vi "Broadcast Map File Path.vi"(8 "error in (no error)":errorcluster, 11 "Yaml Model in":refnum<class "Yaml Model.lvclass">) -> (0 "error out":errorcluster, 3 "Yaml Model out":refnum<class "Yaml Model.lvclass">)   [LabVIEW 2020, in "Yaml Model.lvlib" / "Yaml Model.lvclass"]
uses:
  Yaml Model.lvclass
  Yaml Model Messages/Abstract Map File Path Msg/Abstract Map File Path Msg.lvclass
  C:/Program Files/National Instruments/LabVIEW 2020/vi.lib/ActorFrameworkObserver/Data Message/Data Message.lvclass
  Yaml Model.lvclass/Yaml Model.ctl
  <vilib>/ActorFrameworkObserver/Actor Register/Actor Register.lvclass
panel:
  # "NOTICE -- YOU MUST LEAVE THIS NOTICE IN PLACE.\n\nCopyright (c) 2017, LIANG LIU Shawn.Liu.cn@gmail.com\nAll rights reserved.\n\nRedistribution and use in source and binary forms, with or without modification, are permitted provided that the following conditions are met:\n-Redistributions of source code must retain the above copyright notice, this list of conditions and the following disclaimer.\n-Redistributions in binary form must reproduce the above copyright notice, this list of conditions and the following disclaimer in the documentation and/or other materials provided with the distribution.\n-Neither the name of the eLp nor the names of its contributors may be used to endorse or promote products derived from this software without specific prior written permission.\n\nTHIS SOFTWARE IS PROVIDED BY THE COPYRIGHT HOLDERS AND CONTRIBUTORS \"AS IS\" AND ANY EXPRESS OR IMPLIED WARRANTIES, INCLUDING, BUT NOT LIMITED TO, THE IMPLIED WARRANTIES OF MERCHANTABILITY AND FITNESS FOR A PARTICULAR PURPOSE ARE DISCLAIMED. IN NO EVENT SHALL THE COPYRIGHT HOLDER OR CONTRIBUTORS BE LIABLE FOR ANY DIRECT, INDIRECT, INCIDENTAL, SPECIAL, EXEMPLARY, OR CONSEQUENTIAL DAMAGES (INCLUDING, BUT NOT LIMITED TO, PROCUREMENT OF SUBSTITUTE GOODS OR SERVICES; LOSS OF USE, DATA, OR PROFITS; OR BUSINESS INTERRUPTION) HOWEVER CAUSED AND ON ANY THEORY OF LIABILITY, WHETHER IN CONTRACT, STRICT LIABILITY, OR TORT (INCLUDING NEGLIGENCE OR OTHERWISE) ARISING IN ANY WAY OUT OF THE USE OF THIS SOFTWARE, EVEN IF ADVISED OF THE POSSIBILITY OF SUCH DAMAGE."
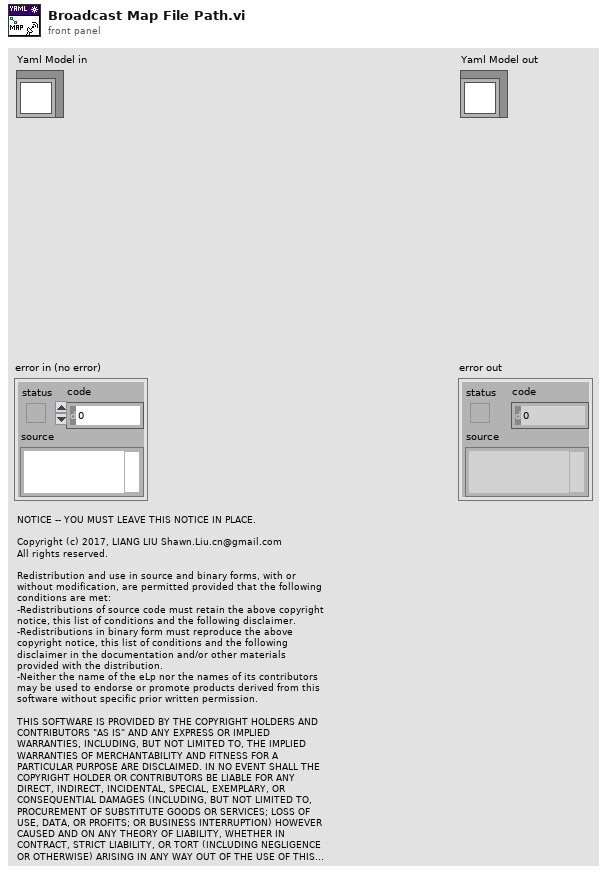
[diagram p1: front panel]
types:
  T1 = cluster{"Image":string, "Resolution":dbl, "Origin":cluster{"X":dbl, "Y":dbl, "R":dbl}, "Occupied Thresh":dbl, "Free Thresh":dbl, "Negate":bool}
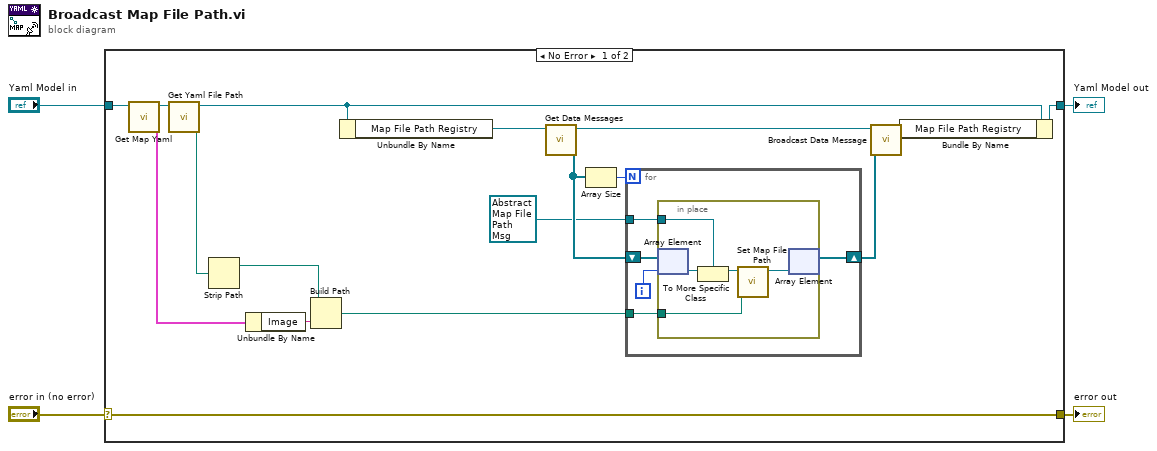
[diagram p0: block diagram]
diagram:
  n1 = case shown="No Error" "error in (no error)" {
    selector: "error in (no error)" -> [w19 w33]
    tunnel: "Yaml Model in" -> [w21 w32]
    tunnel: [w20 w32] -> w3
    tunnel: [w19 w33] -> w1
    frame No Error {
      n2 = call "Get Map Yaml.vi"("Yaml Model in"=w21) -> ("Map Yaml"=w14:T1, "Yaml Model out"=w18:refnum<class "Yaml Model.lvclass">)  [unwired: 9 in]
      n3 = call "Get Yaml File Path.vi"("Yaml Model in"=w18) -> ("Yaml File Path"=w16:path, "Yaml Model out"=w17:refnum<class "Yaml Model.lvclass">)  [unwired: 9 in]
      n4 = Strip Path(path=w16) -> (stripped path=w15:path)  [unwired: 1 out]
      n5 = Unbundle By Name(w14) -> ("Image"=w13:string)
      n6 = Build Path(base path=w15, name or relative path=w13) -> (appended path=w5:path)
      n7 = Unbundle By Name(w17) -> ("Map File Path Registry"=w12:refnum<class "Actor Register.lvclass">)
      n8 = call-dynamic "Get Data Messages.vi"("Actor Register in"=w12) -> ("Data Messages"=w9:refnum<class "Data Message.lvclass">[], "Actor Register out"=w11:refnum<class "Actor Register.lvclass">)  [unwired: 9 in]
      n9 = Array Size(array=w9) -> (size(s)=w7:i32)
      n10 = for {
        N: w7 -> [_]
        shift-right: [w24] -> w6
        shift-left: w9 -> [w26]
        tunnel: refnum<class "Abstract Map File Path Msg.lvclass"> refnum ("Yaml Model.lvlib:Abstract Map File Path Msg.lvclass") -> [w25]
        tunnel: w5 -> [w22]
        i -> [w23]
        n11 = in-place {
          in-place-border: w25 -> [w30]
          in-place-border: w22 -> [w27]
          n12 = in-place-array #1(w26, w23) -> (w31:refnum<class "Data Message.lvclass">)
          n13 = To More Specific Class(target class=w30, reference=w31) -> (specific class reference=w29:refnum<class "Abstract Map File Path Msg.lvclass">)  [unwired: 1 in, 1 out]
          n14 = call "Set Map File Path.vi"("Map File Path"=w27, "Abstract Map File Path Msg in"=w29) -> ("Abstract Map File Path Msg out"=w28:refnum<class "Abstract Map File Path Msg.lvclass">)  [unwired: 9 in]
          n15 = in-place-array #1(w28) -> (w24:refnum<class "Data Message.lvclass">[])  [unwired: 1 out]
        }
      }
      n16 = call <vilib>:"Broadcast Data Message.vi"("Data Messages"=w6, "Actor Register in"=w11) -> ("Actor Register out"=w10:refnum<class "Actor Register.lvclass">)  [unwired: 8 in, 1 out]
      n17 = Bundle By Name(cluster=w17, "Map File Path Registry"=w10) -> (w20:refnum<class "Yaml Model.lvclass">)
    }
    frame Error {
    }
  }
  "error out" <- w1
  "Yaml Model out" <- w3
